vi "ma_Compute t0 eps timestamp.vi"(10 "t0 entry":timestamp format="%<%.4X>T") -> (3 "t0 eps":dbl format="%0.6e")   [LabVIEW 2022 SP3, in "NI_MABase.lvlib"]
uses:
  NI_MABase.lvlib
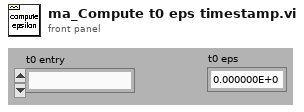
[diagram p1: front panel]
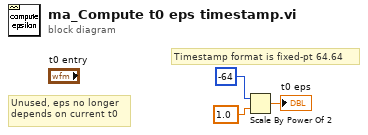
[diagram p0: block diagram]
diagram:
  # "Unused, eps no longer\ndepends on current t0"
  # "Timestamp format is fixed-pt 64.64"
  n1 = Scale By Power Of 2(n=-64 ("x"), x=1.0) -> (x*2^n=→"t0 eps":dbl)
